vi "Test gRPC Timing - Automatic Launch.vi"   [LabVIEW 2021]
uses:
  gRPC/test_service_server/test_service_server.lvlib
panel:
  # "<<< Note that this\ndoesn't shut down\nthe gRPC server which\nhas its own stop button"
types:
  T1 = typedef "TYPEDEF - Overall Timing Statistics.ctl" = cluster{"Mean Time (usec)":dbl, "Min Time (usec)":dbl, "Max Time (usec)":dbl, "Std Dev (usec)":dbl}
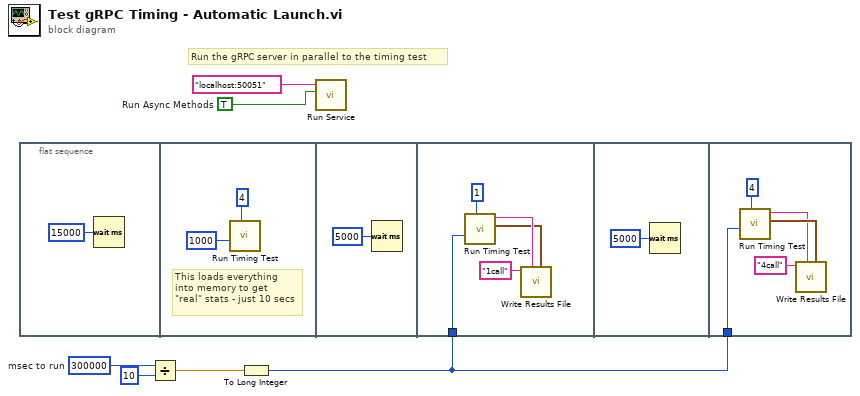
[diagram p0: block diagram]
diagram:
  w4 = 300000  # msec to run
  w6 = TRUE  # Run Async Methods
  # "Run the gRPC server in parallel to the timing test"
  n1 = flat-sequence {
    tunnel: w1 -> [w14]
    tunnel: w1 -> [w17]
    frame #0 {
      n2 = Wait (ms)(milliseconds to wait=u32 15000) -> ()  [unwired: 1 out]
    }
    frame #1 {
      # "This loads everything\ninto memory to get\n\"real\" stats - just 10 secs"
      n3 = call "Run Timing Test.vi"("Number of Concurrent Calls (4)"=4, "Number of Iterations (12000)"=1000) -> ()  [unwired: 7 in, 3 out]
    }
    frame #2 {
      n4 = Wait (ms)(milliseconds to wait=u32 5000) -> ()  [unwired: 1 out]
    }
    frame #3 {
      n5 = call "Run Timing Test.vi"("Number of Concurrent Calls (4)"=1, "Number of Iterations (12000)"=w14) -> ("Timing Stats"=w12:T1, "All Roundtrip Measurments (usec)"=w13:string)  [unwired: 7 in, 1 out]
      n6 = call "Write Results File.vi"("Timing Stats"=w12, "All Roundtrip Measurments (usec)"=w13, "Filename"="1call") -> ()  [unwired: 8 in, 1 out]
    }
    frame #4 {
      n7 = Wait (ms)(milliseconds to wait=u32 5000) -> ()  [unwired: 1 out]
    }
    frame #5 {
      n8 = call "Run Timing Test.vi"("Number of Concurrent Calls (4)"=4, "Number of Iterations (12000)"=w17) -> ("Timing Stats"=w20:T1, "All Roundtrip Measurments (usec)"=w19:string)  [unwired: 7 in, 1 out]
      n9 = call "Write Results File.vi"("Timing Stats"=w20, "All Roundtrip Measurments (usec)"=w19, "Filename"="4call") -> ()  [unwired: 8 in, 1 out]
    }
  }
  n10 = Divide(x=w4, y=10) -> (x/y=w3:dbl)
  n11 = To Long Integer(number=w3) -> (32bit integer=w1:i32)
  n12 = call "Run Service.vi"("Async [T] / Sync [F]"=w6, "Server Address"="localhost:50051") -> ()  [unwired: 10 in]
